vi "Clear Alarm.vi"(8 "error in (no error)":errorcluster, 10 "Alarm Code":i32, 11 "Alarm Handler Actor in":refnum<class "Alarm Handler Actor.lvclass">) -> (0 "error out":errorcluster, 3 "Alarm Handler Actor out":refnum<class "Alarm Handler Actor.lvclass">)   [LabVIEW 2015, in "Alarm Handler Actor.lvclass"]
doc: "Searches through the Active Alarms and removes the <b>Alarm</b> if it is found. Additionally this clear action is logged.\n\nIf the <b>Alarm</b> is not active then no further action is taken."
uses:
  Alarm Handler Actor.lvclass
  Alarm Handler Actor.lvclass/Alarm Handler Actor.ctl
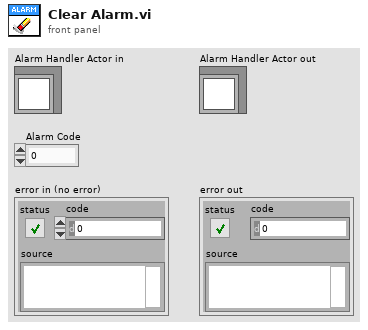
[diagram p1: front panel]
types:
  T1 = typedef "Alarm Handler Actor.lvclass/Active Alarm.ctl" = cluster{"Alarm Detail":T2, "Count":i32, "First Error":timestamp, "Last Error":timestamp, "LabVIEW Error":bool}
  T2 = typedef "Alarm Handler Actor.lvclass/Alarm Details.ctl" = cluster{"Code":i32, "Loop":i32, "Description":string, "Severity":i32, "Clear on Ack?":bool, "Log All Events?":bool}
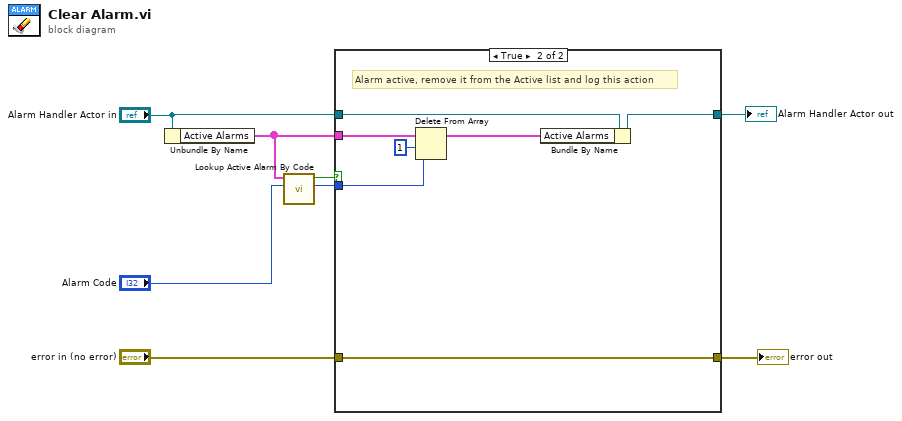
[diagram p0: block diagram]
diagram:
  n1 = Unbundle By Name("Alarm Handler Actor in") -> ("Active Alarms"=w4:T1[])
  n2 = call "Lookup Active Alarm By Code.vi"("Code"="Alarm Code", "Active Alarms"=w4) -> ("Index"=w2:i32, "Found"=w3:bool)  [unwired: 8 in]
  n3 = case shown="True" w3 {
    tunnel: "error in (no error)" -> [w9 w11]
    tunnel: [w9 w11] -> w7
    tunnel: [w10 w14] -> w6
    tunnel: "Alarm Handler Actor in" -> [w10 w15]
    tunnel: w2 -> [_ w12]
    tunnel: w4 -> [_ w17]
    frame False {
      # "Alarm not actually active, do nothing"
    }
    frame True {
      # "Alarm active, remove it from the Active list and log this action"
      n4 = Delete From Array(array=w17, length=1, index=w12) -> (array with subset deleted=w13:T1[])  [unwired: 1 out]
      n5 = Bundle By Name(cluster=w15, "Active Alarms"=w13) -> (w14:refnum<class "Alarm Handler Actor.lvclass">)
    }
  }
  "error out" <- w7
  "Alarm Handler Actor out" <- w6
